vi "Test Customer with Phone Finishing Call Broadcasts Status.vi"(8 "error in (no error)":errorcluster, 11 "Customer With Phone Test In":refnum<class "Customer With Phone Test.lvclass">) -> (0 "error out":errorcluster, 3 "Customer With Phone Test Out":refnum<class "Customer With Phone Test.lvclass">)   [LabVIEW 2020, in "Customer With Phone Test.lvclass"]
uses:
  Customer With Phone Test.lvclass
  C:/Program Files (x86)/National Instruments/LabVIEW 2020/vi.lib/Asteme/LUnit/Test Case.lvclass
  Processes/People/Customers/Customer With Phone/Customer With Phone.lvclass
  C:/Program Files (x86)/National Instruments/LabVIEW 2020/vi.lib/Asteme/Triarc Framework/Process/Process.lvclass
  <vilib>/Asteme/Triarc Framework/Process/Process.lvclass/Process.ctl
  <vilib>/Asteme/LUnit/Test Case.lvclass/Test Case.ctl
  <vilib>/Asteme/LUnit/LUnit Assertion Result.lvclass/LUnit Assertion Result.ctl
  <vilib>/Asteme/Triarc Framework/Broadcast Event Helpers/Execution timer.vi
  <vilib>/Asteme/Triarc Framework/Process/Private/SubVIs/Wait for finish.vi
  <vilib>/Asteme/Triarc Framework/Process/Protected/Messaging/Enqueue Message.vi
  <vilib>/Asteme/Triarc Framework/Process/Private/SubVIs/Set Lifecycle State.vi
  <vilib>/Asteme/Triarc Framework/Process/Public/Lifecycle/Get Lifecycle State.vi
  <vilib>/Asteme/LUnit/Palette/Pass.vi
  <vilib>/Asteme/LUnit/Palette/Fail.vi
  <vilib>/Asteme/LUnit/Variant to string.vi
  <vilib>/Asteme/LUnit/Set Assertion Type.vi
  <vilib>/Utility/error.llb/Clear Errors.vi
  <vilib>/Asteme/LUnit/Add test result.vi
  <vilib>/Asteme/LUnit/LUnit Write Passed.vi
  <vilib>/Asteme/LUnit/LUnit Get Test Case.vi
  <vilib>/Asteme/LUnit/Assertion Result/LUnit Get Test Name.vi
  <vilib>/Asteme/LUnit/LUnit Write Message.vi
  <vilib>/Asteme/LUnit/LUnit Write Description.vi
  <vilib>/Asteme/LUnit/LUnit Write Assertion Type.vi
  <vilib>/Asteme/LUnit/Read Test Case Name.vi
  <vilib>/Asteme/Triarc Framework/Broadcast Event Helpers/Dequeue Broadcast Message.vi
  <vilib>/Utility/error.llb/Error Cluster From Error Code.vi
  <vilib>/Utility/Data Type/Get Type Information.vi
  <vilib>/Utility/LVClass/Get LV Class Name.vi
  <vilib>/Asteme/LUnit/LUnit Assertion Result.lvclass
  <vilib>/Asteme/Triarc Framework/Process/Process.lvclass
  <vilib>/Asteme/LUnit/Test Case.lvclass
  <vilib>/Asteme/Triarc Framework/Broadcast Event Helpers/Broadcast Event Helpers.lvlib
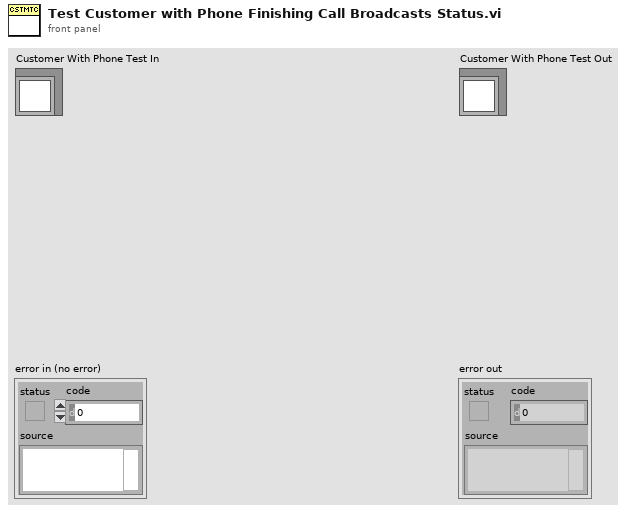
[diagram p1: front panel]
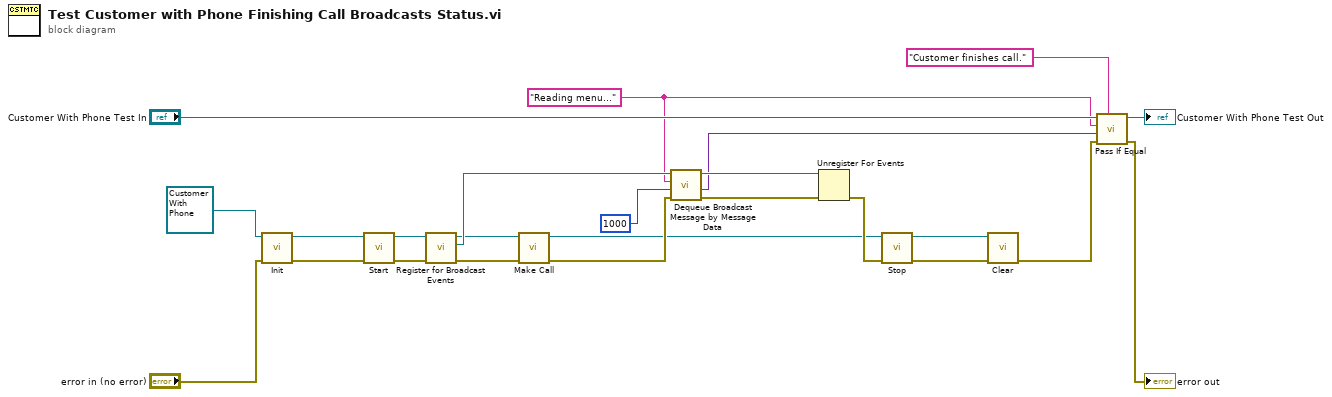
[diagram p0: block diagram]
diagram:
  w1 = "Reading menu..."
  n1 = call-dynamic "Init.vi"("error in (no error)"="error in (no error)", "View In"=refnum<class "Customer With Phone.lvclass"> refnum ("Customer With Phone.lvclass")) -> ("error out"=w24:errorcluster, "View Out"=w13:refnum<class "Customer With Phone.lvclass">)  [unwired: 8 in]
  n2 = call <vilib>:"Start.vi"("error in (no error)"=w24, "Process In"=w13) -> ("error out"=w16:errorcluster, "Process Out"=w18:refnum<class "Customer With Phone.lvclass">)  [unwired: 8 in]
  n3 = call <vilib>:"Register for Broadcast Events.vi"("error in (no error)"=w16, "Process In"=w18) -> ("error out"=w17:errorcluster, "Event Registration Refnum Out"=w22:refnum<event-registration>, "Process Out"=w19:refnum<class "Customer With Phone.lvclass">)  [unwired: 7 in]
  n4 = call "Make Call.vi"("error in (no error)"=w17, "Customer With Phone In"=w19) -> ("error out"=w21:errorcluster, "Customer With Phone Out"=w20:refnum<class "Customer With Phone.lvclass">)  [unwired: 8 in]
  n5 = call <vilib>:"Dequeue Broadcast Message by Message Data.vi"("error in (no error)"=w21, "Timeout (-1)"=1000, "Message Data"=w1, "Event Registration Refnum"=w22) -> ("error out"=w4:errorcluster, "Message Data"=w2:variant, "Event Registration Refnum Out"=w5:refnum<event-registration>)  [unwired: 3 in, 2 out]
  n6 = Unregister For Events(event registration refnum=w5, error in=w4) -> (error out=w23:errorcluster)
  n7 = call <vilib>:"Stop.vi"("error in (no error)"=w23, "Process In"=w20) -> ("error out"=w15:errorcluster, "Process Out"=w14:refnum<class "Customer With Phone.lvclass">)  [unwired: 7 in, 1 out]
  n8 = call-dynamic "Clear.vi"("error in (no error)"=w15, "View In"=w14) -> ("error out"=w7:errorcluster)  [unwired: 9 in]
  n9 = call <vilib>:"Pass If Equal.vi"("Description"="Customer finishes call.", "error in (no error)"=w7, "Actual"=w2, "Expected"=w1, "Test Case In"="Customer With Phone Test In") -> ("error out"=→"error out":errorcluster, "Test Case Out"=→"Customer With Phone Test Out":refnum<class "Customer With Phone Test.lvclass">)  [unwired: 5 in]
